vi "FGV_USER_EDITOR_records_display.vi"(4 "front_panel_reference":refnum<vi>, 6 "SQL_listbox_reference":refnum<vi>, 7 "options":T3, 8 "error_in":errorcluster, 10 "uneditable_columns":string[](array[string]), 11 "input":variant) -> (0 "error_out":errorcluster, 1 "all_info":T1, 2 "array_param_output":string[](array[string]), 3 "string_param_output":string)   [LabVIEW 2019]
uses:
  FGV_USER_EDITOR_records_display.ctl
  USER_EDITOR_all_info.ctl
  MAIN/SQL_record_states.ctl
  ini/typedef/CLIENT_all_config_info.ctl
  ini/typedef/CLIENT_main_ini_file.ctl
  queues/typedef/CLIENT_queue_refnums.ctl
  queues/typedef/SQL_EDITOR_queue_element.ctl
  MAIN/SQL_EDITOR/SQL_EDITOR_sequence_state.ctl
  queues/typedef/CLIENT_SCANNER_queue_element.ctl
  MAIN/SCANNER/SCANNER_sequence_state.ctl
  queues/typedef/CLIENT_REF_CHG_queue_element.ctl
  MAIN/reference_changed_connection/CLIENT_REF_CHG_sequence_state.ctl
  login/FGV_login.ctl
  <userlib>/_OpenG.lib/array/array.llb/Filter 1D Array (String)__ogtk.vi
  <userlib>/_OpenG.lib/array/array.llb/Delete Elements from 1D Array (I32)__ogtk.vi
  <vilib>/addons/database/_DB Variant To Data/Database Variant To Data.xnode
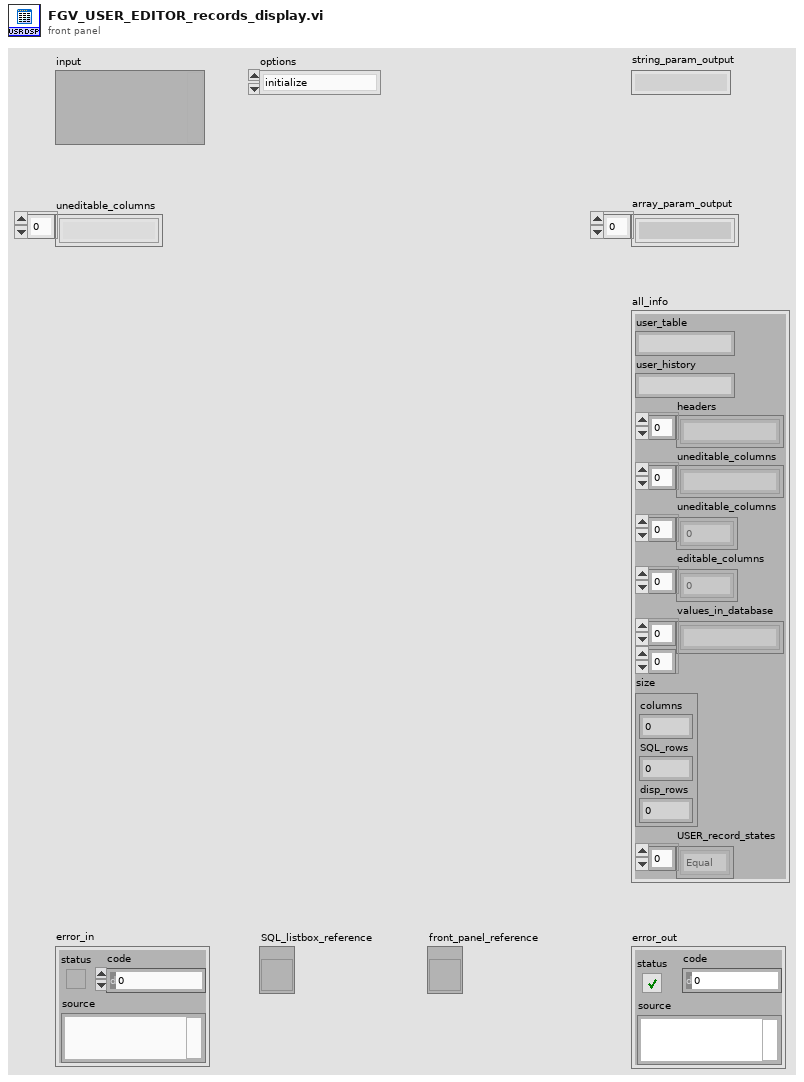
[diagram p1: front panel]
types:
  T1 = typedef "USER_EDITOR_all_info.ctl" = cluster{"user_table":string, "user_history":string, "headers":string[], "uneditable_columns":string[], "uneditable_columns":i32[], "editable_columns":i32[], "values_in_database":string[][], "size":cluster{"columns":i32, "SQL_rows":i32, "disp_rows":i32}, "USER_record_states":T2[]}
  T2 = typedef "SQL_record_states.ctl" = enum16{"Equal", "Added", "Edited", "Deleted"}
  T3 = typedef "FGV_USER_EDITOR_records_display.ctl" = enum16{"initialize", "set_user_edit_tables_names", "set_headers", "set_records", "get_user_edit_table_name", "get_user_edit_hist_table_name", "get_headers", "get_uneditable_columns", "get_all_info", "record_added?", "record_inserted?", "record_edited?", "record_updated?", "record_deleted?", "discard_changes"}
  T4 = typedef "CLIENT_all_config_info.ctl" = cluster{"main_ini_file":T5, "SQL Password":string, "queue_refnums":T6}
  T5 = typedef "CLIENT_main_ini_file.ctl" = cluster{"SQL Driver":string, "SQL Server":string, "SQL Database":string, "SQL UID":string, "Reference table":string, "Reference history":string, "Archivisation CFG table":string, "Archivisation CFG history":string, "User table":string, "User history":string, "logout timeout [ms]":i32, "records per page":i32, "default language":string, "REF CHG connection IP":string, "REF CHG remote port":i32, "REF CHG local port":i32, "SCANNER COM port":u16, "SCANNER Baud rate":u32, "SCANNER Data bits":u16, "SCANNER Pairity":enum16{"None", "Odd", "Even", "Mark", "Space"}, "SCANNER Stop bits":u16, "SCANNER Flow control":u16, "SCANNER Termination char":u8}
  T6 = typedef "CLIENT_queue_refnums.ctl" = cluster{"SQL_EDITOR_queue":refnum<queue>, "SCANNER_queue":refnum<queue>, "SCANNER_data":refnum<queue>, "CLIENT_REF_CHG_queue":refnum<queue>}
  T7 = typedef "FGV_login.ctl" = enum16{"initialize", "login", "logout", "get_login_info"}
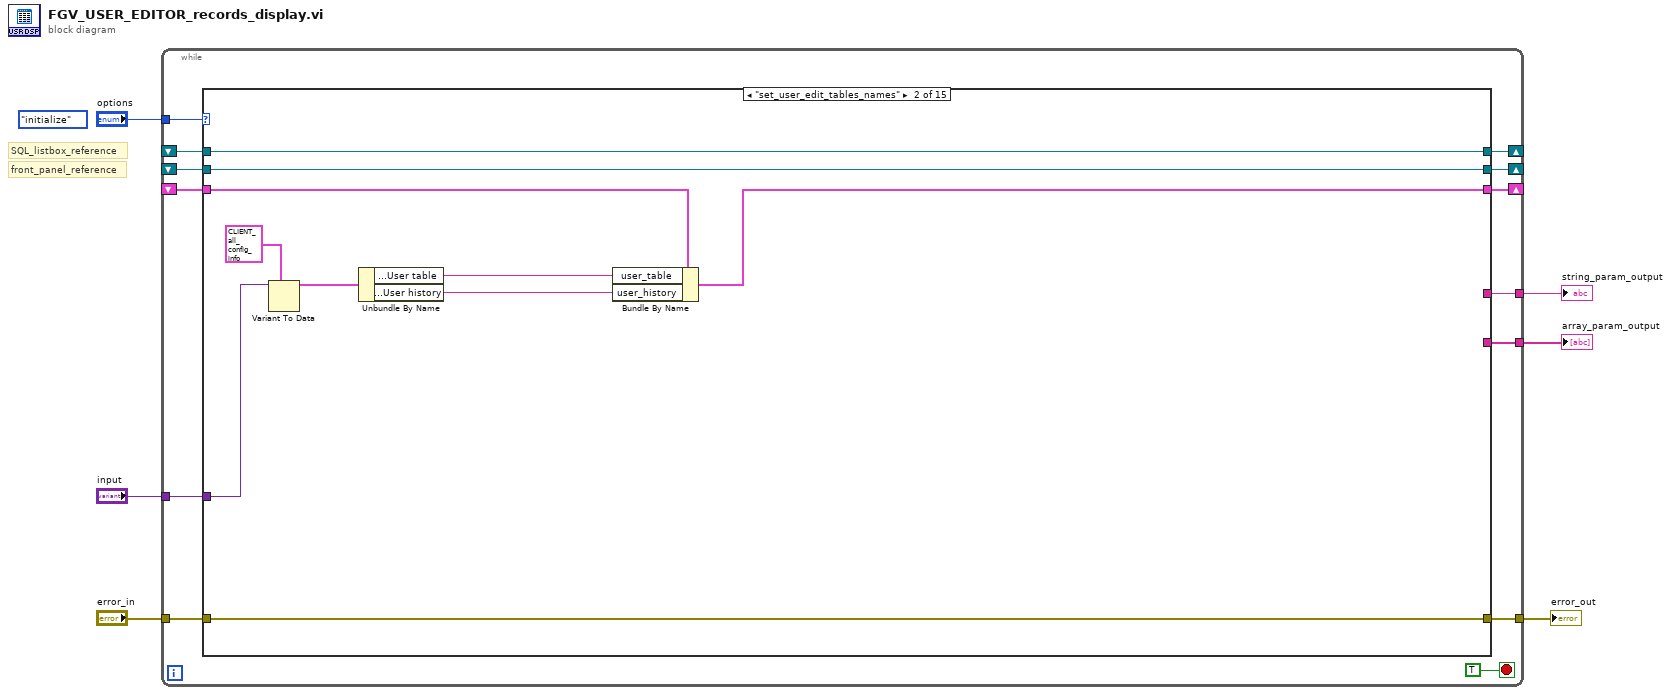
[diagram p0: block diagram]
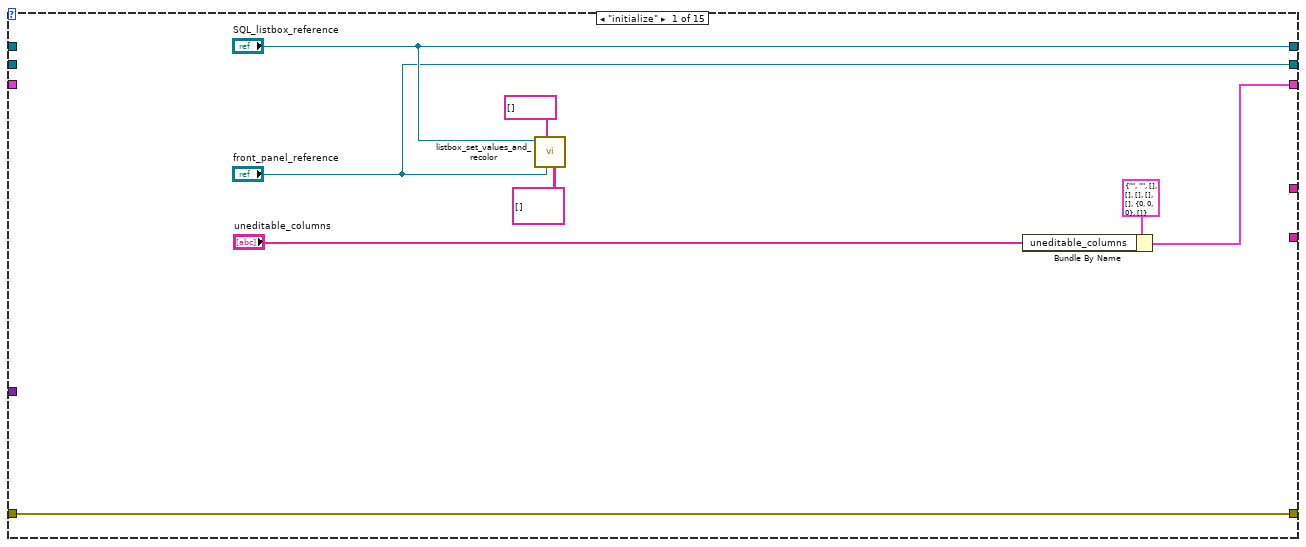
[diagram p2: hidden frame]
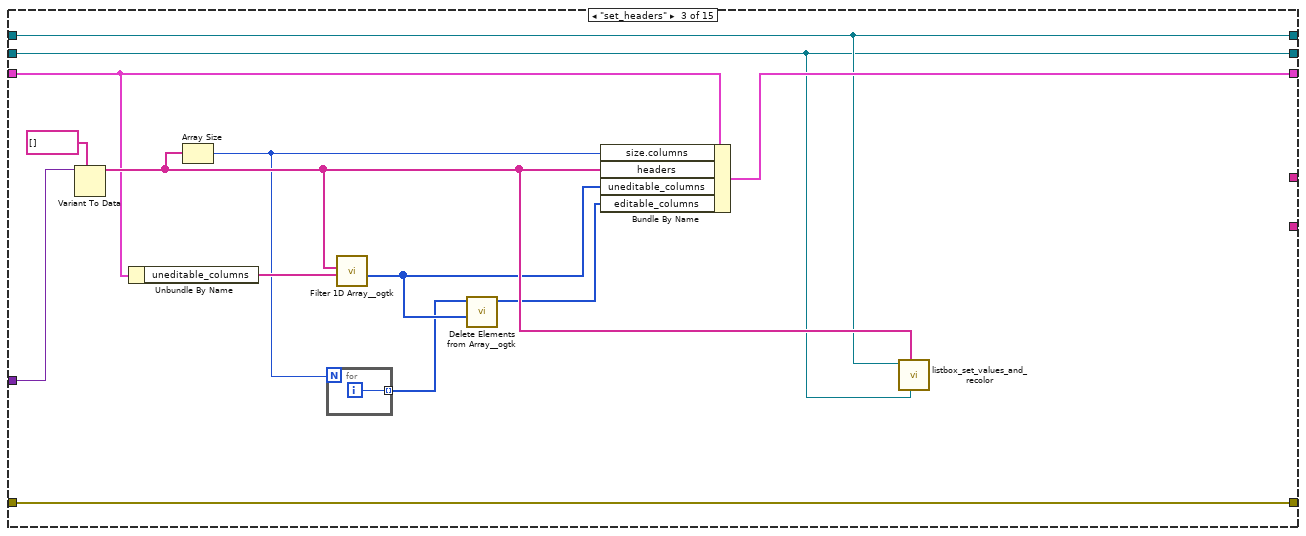
[diagram p3: hidden frame]
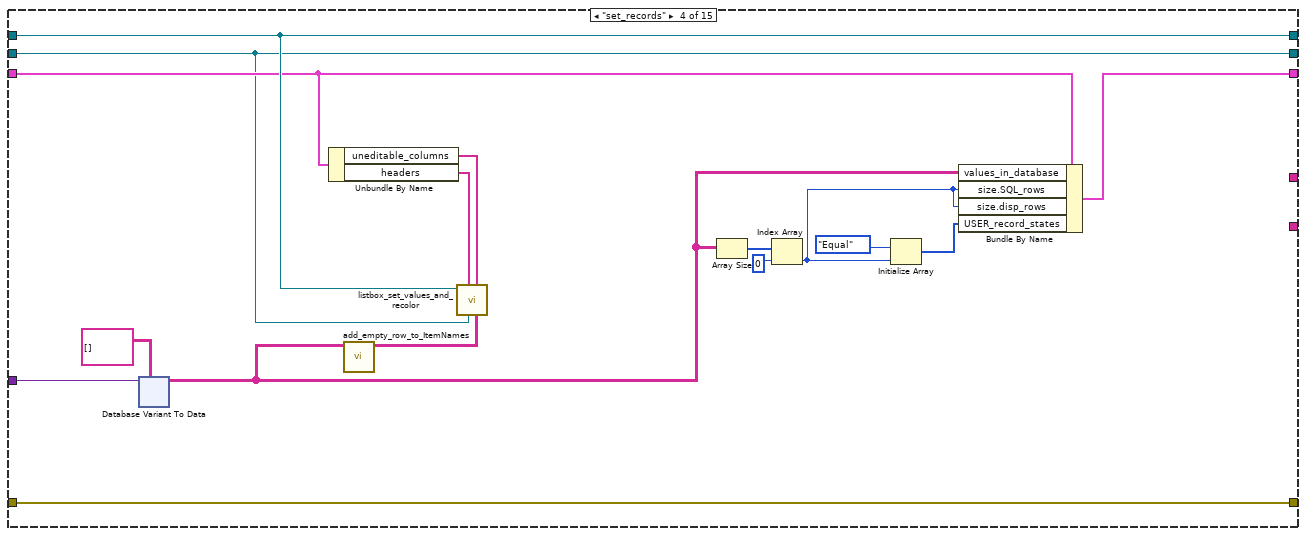
[diagram p4: hidden frame]
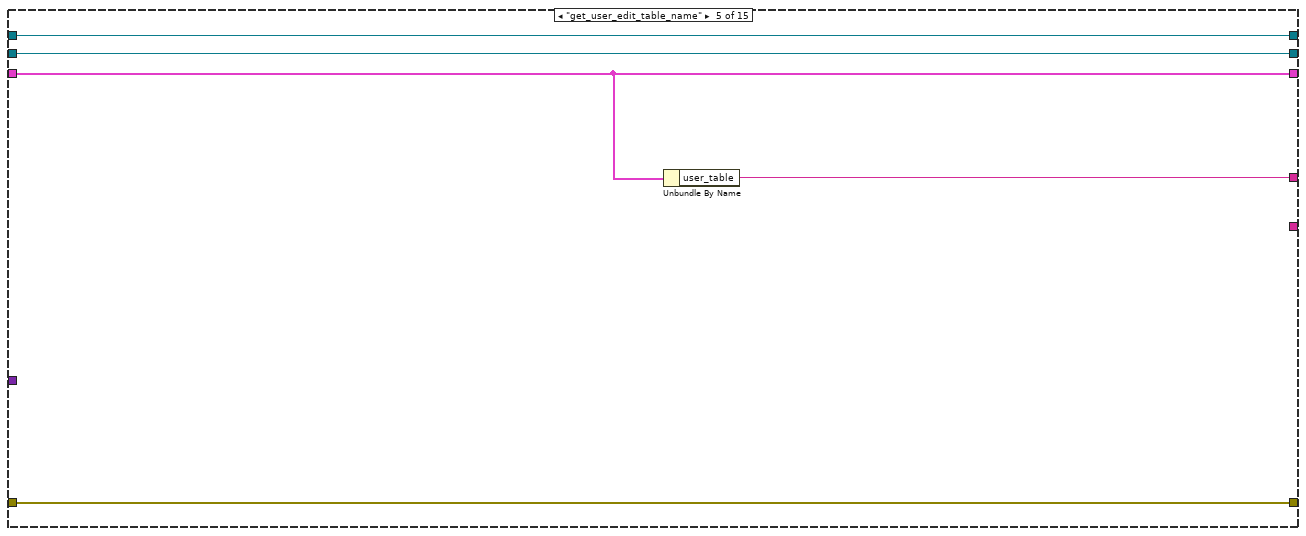
[diagram p5: hidden frame]
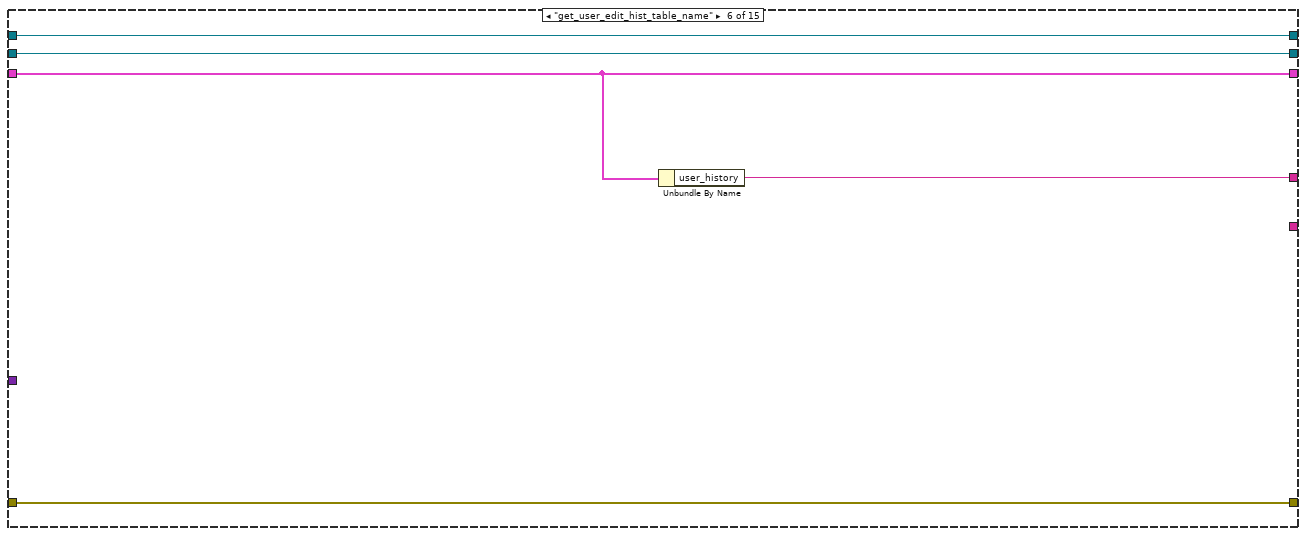
[diagram p6: hidden frame]
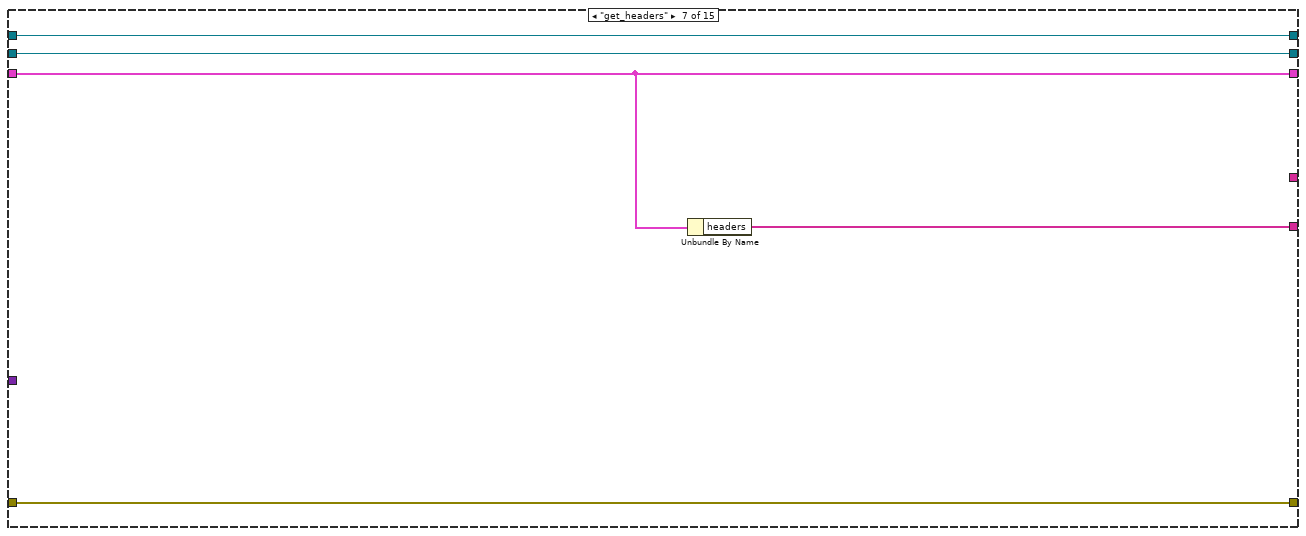
[diagram p7: hidden frame]
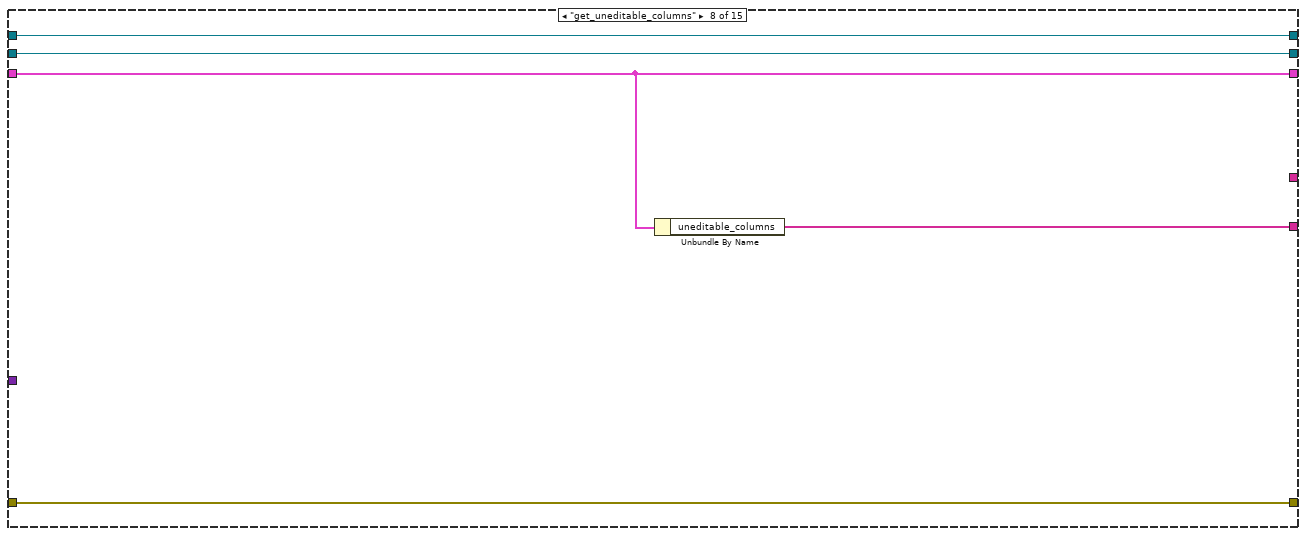
[diagram p8: hidden frame]
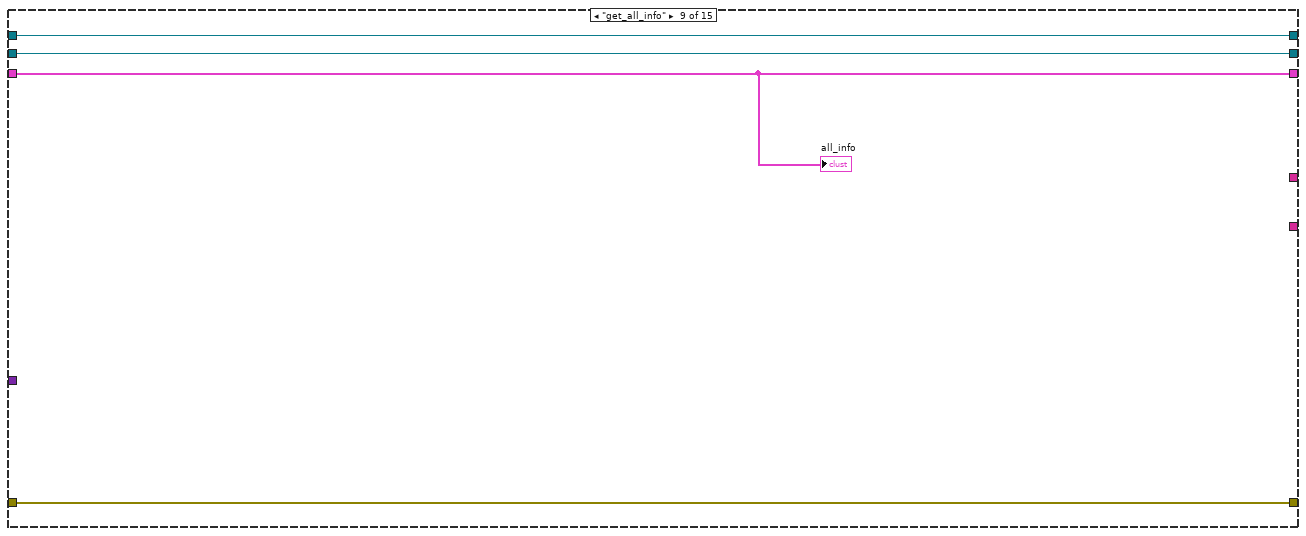
[diagram p9: hidden frame]
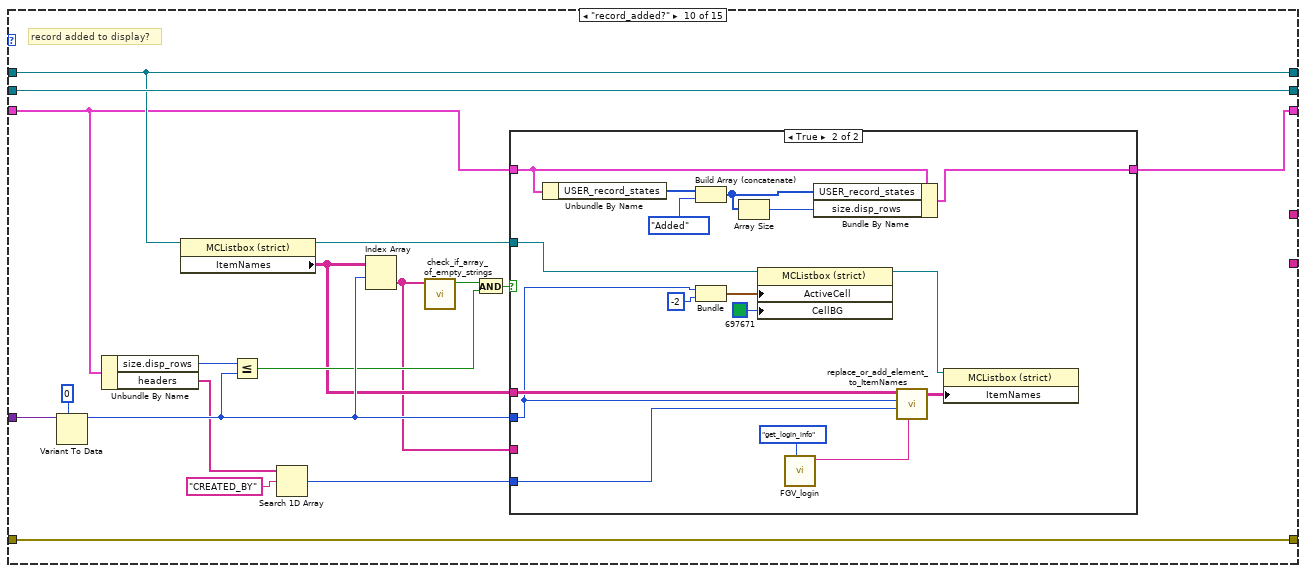
[diagram p10: hidden frame]
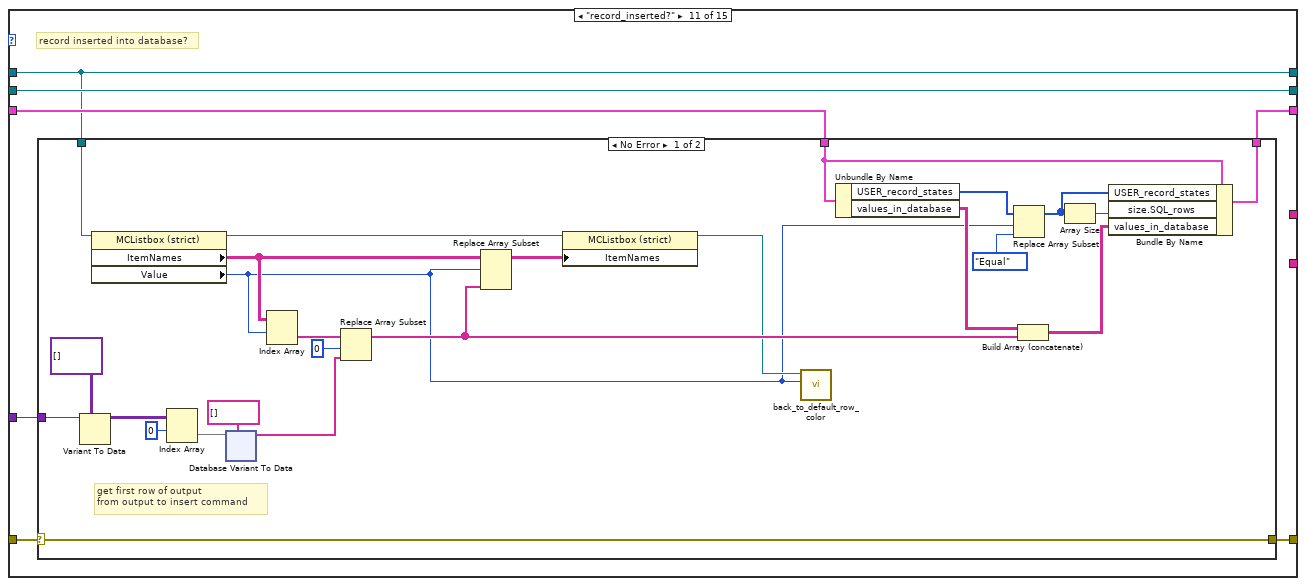
[diagram p12: hidden frame]
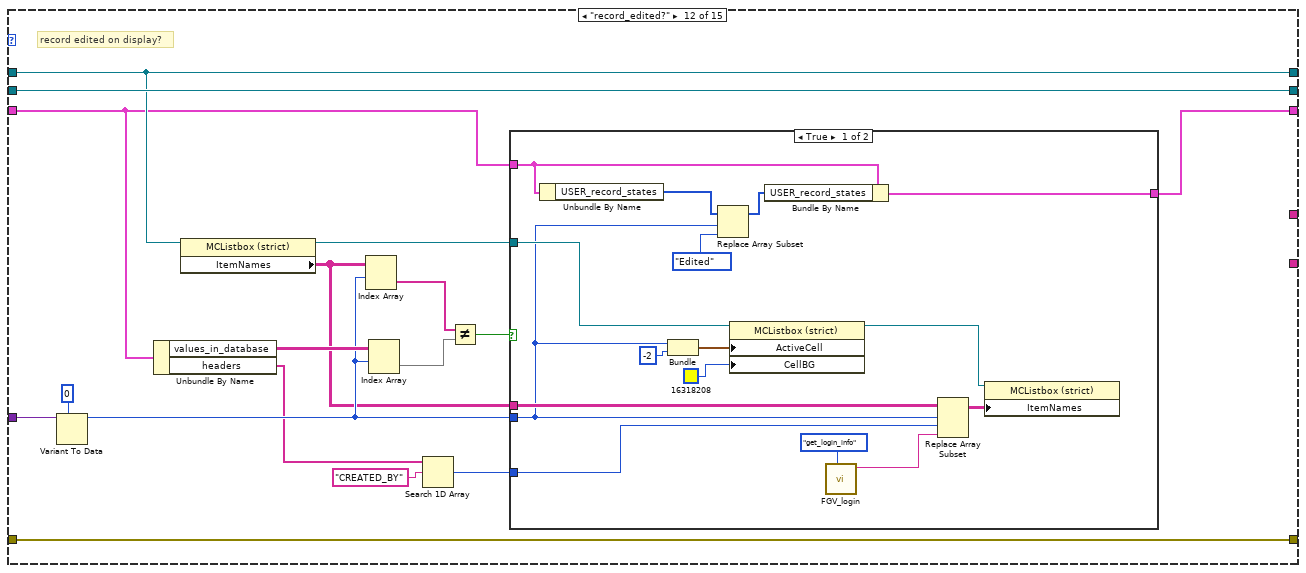
[diagram p14: hidden frame]
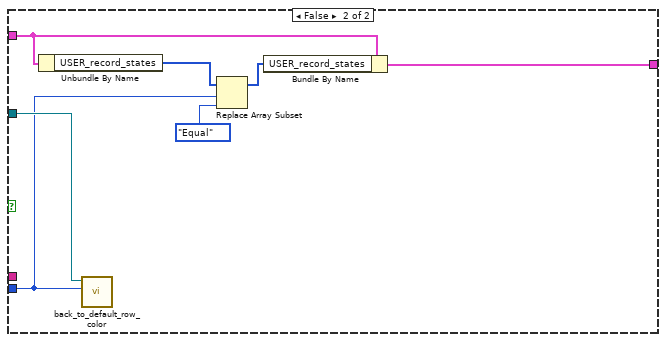
[diagram p15: hidden frame]
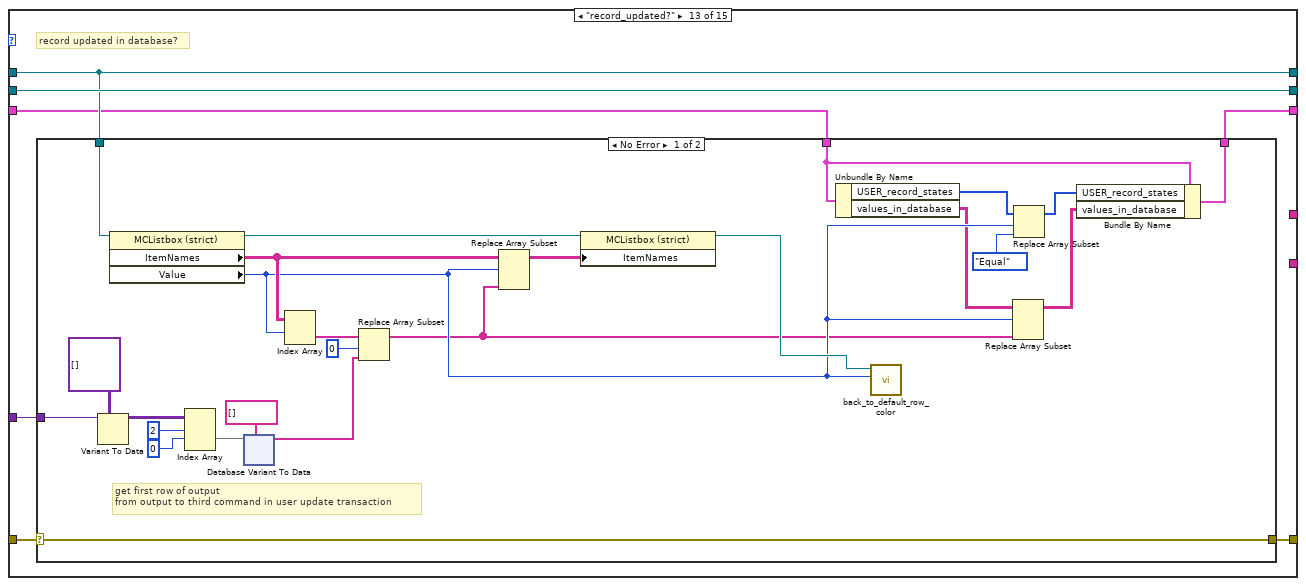
[diagram p16: hidden frame]
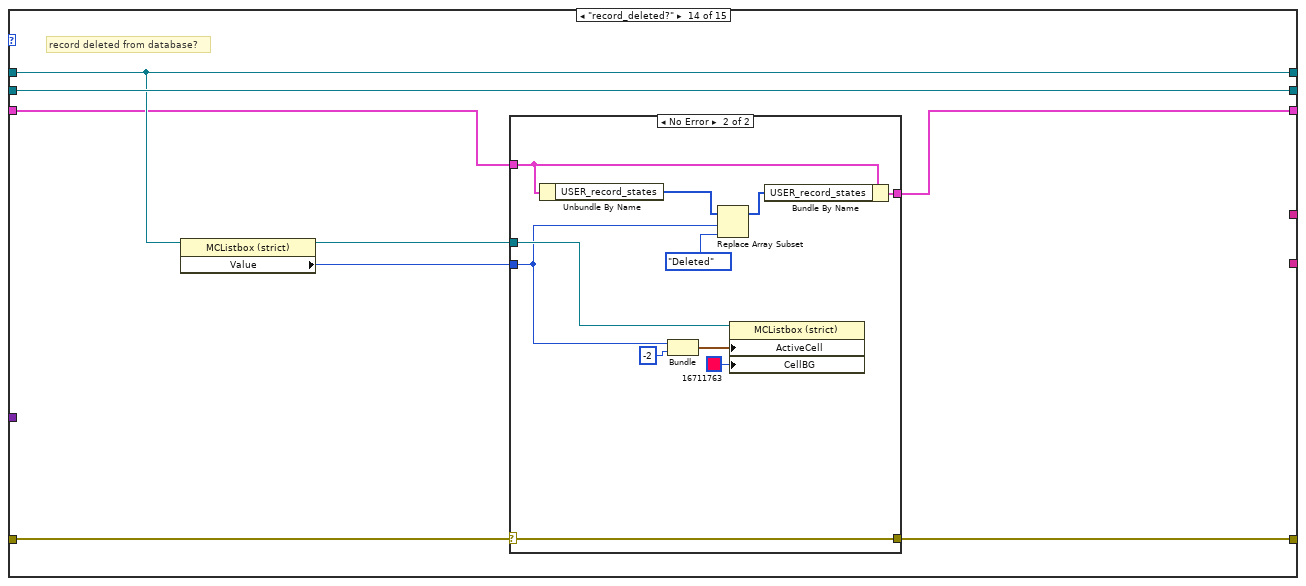
[diagram p18: hidden frame]
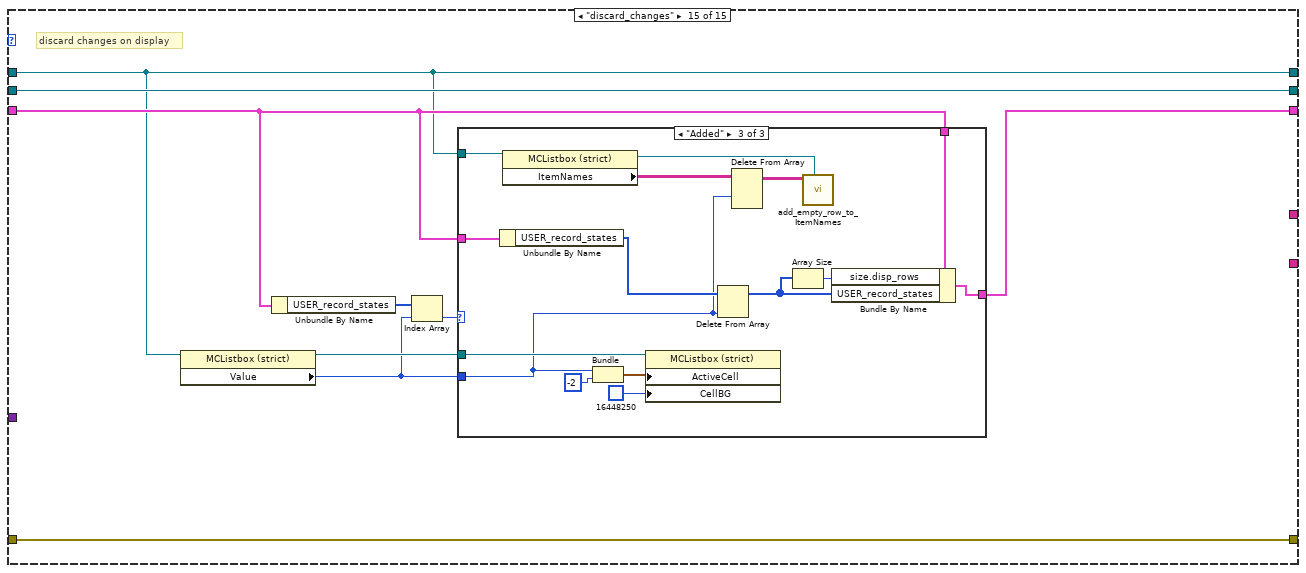
[diagram p20: hidden frame]
diagram:
  (unwired) FGV_USER_EDITOR_records_display."initialize" ("options")
  # "front_panel_reference"
  # "SQL_listbox_reference"
  n1 = while {
    tunnel: "options" -> [w18]
    tunnel: [w17] -> w6
    tunnel: "error_in" -> [w16]
    shift-right: [w15] -> _
    shift-left: _ -> [w14]
    tunnel: [w13] -> w3
    shift-right: [w12] -> _
    shift-left: _ -> [w11]
    tunnel: [w10] -> w2
    tunnel: "input" -> [w9]
    shift-right: [w8] -> _
    shift-left: _ -> [w7]
    stop <- TRUE stop-if-true
    n2 = case shown="\"set_user_edit_tables_names\"" w18 {
      tunnel: [w27 w37 w50 w65 w102 w107 w113 w118 w122 w141 w160 w248 w272 w345 w370] -> w17
      tunnel: w16 -> [w27 w37 w50 w65 w102 w107 w113 w118 w122 w141 w161 w248 w273 w346 w370]
      tunnel: [w23 w35 w40 w61 w104 w109 w114 w119 w123 w135 w164 w236 w275 w347 w371] -> w15
      tunnel: w14 -> [_ w36 w41 w62 w104 w109 w114 w119 w123 w133 w165 w237 w276 w348 w366]
      tunnel: [_ _ _ _ w103 w108 _ _ _ _ _ _ _ _ _] -> w13
      tunnel: ["SQL_listbox_reference" w34 w39 w64 w101 w106 w110 w117 w121 w137 w162 w243 w277 w350 w365] -> w12
      tunnel: w11 -> [_ w34 w39 w64 w101 w106 w110 w117 w121 w137 w162 w243 w277 w350 w365]
      tunnel: [_ _ _ _ _ _ w112 w116 _ _ _ _ _ _ _] -> w10
      tunnel: w9 -> [_ w33 w42 w66 _ _ _ _ _ w139 w163 w246 w274 _ _]
      tunnel: ["front_panel_reference" w32 w38 w54 w100 w105 w111 w115 w120 w140 w166 w247 w278 w351 w373] -> w8
      tunnel: w7 -> [_ w32 w38 w54 w100 w105 w111 w115 w120 w140 w166 w247 w278 w351 w373]
      frame "initialize" {
        n3 = call "listbox_set_values_and_recolor.vi"("item_names"=string[][] [], "front_panel_reference"="front_panel_reference", "column_names"=string[] [], "multicolumn_listbox_reference_in"="SQL_listbox_reference") -> ()  [unwired: 6 in, 2 out]
        n4 = Bundle By Name(cluster=T1 {"user_table"="", "user_history"="", "headers"=[], "uneditable_columns"=[], "uneditable_columns"=[], "editable_columns"=[], "values_in_database"=[], "size"={"columns"=0, "SQL_rows"=0, "disp_rows"=0}, "USER_record_states"=[]} ("SQL_selection"), "uneditable_columns"="uneditable_columns") -> (w23:T1)
      }
      frame "set_user_edit_tables_names" {
        n5 = Variant To Data(type=T4 {"main_ini_file"={"SQL Driver"="", "SQL Server"="", "SQL Database"="", "SQL UID"="", "Reference table"="", "Reference history"="", "Archivisation CFG table"="", "Archivisation CFG history"="", "User table"="", "User history"="", "logout timeout [ms]"=0, "records per page"=0, "default language"="", "REF CHG connection IP"="", "REF CHG remote port"=0, "REF CHG local port"=0, "SCANNER COM port"=0, "SCANNER Baud rate"=0, "SCANNER Data bits"=0, "SCANNER Pairity"=enum."None", "SCANNER Stop bits"=10, "SCANNER Flow control"=0, "SCANNER Termination char"=0}, "SQL Password"="", "queue_refnums"={"SQL_EDITOR_queue"=refnum, "SCANNER_queue"=refnum, "SCANNER_data"=refnum, "CLIENT_REF_CHG_queue"=refnum}} ("all_config_info"), Variant=w33) -> (data=w31:T4)  [unwired: 1 in, 1 out]
        n6 = Unbundle By Name(w31) -> ("main_ini_file.User table"=w30:string, "main_ini_file.User history"=w29:string)
        n7 = Bundle By Name(cluster=w36, "user_table"=w30, "user_history"=w29) -> (w35:T1)
      }
      frame "set_headers" {
        n8 = Variant To Data(type=string[] [], Variant=w42) -> (data=w48:string[])  [unwired: 1 in, 1 out]
        n9 = Unbundle By Name(w41) -> ("uneditable_columns"=w46:string[])
        n10 = Array Size(array=w48) -> (size(s)=w43:i32)
        n11 = for {
          N: w43 -> [_]
          tunnel: [w51] -> w45 mode=indexing
          i -> [w51]
        }
        n12 = call-poly <userlib>:"Filter 1D Array__ogtk.vi"("items to filter"=w46, "array"=w48) -> ("filtered item indices"=w47:i32[])  [unwired: 4 in, 1 out]
        n13 = call-poly <userlib>:"Delete Elements from Array__ogtk.vi"("indices"=w47, "array"=w45) -> ("array w/ subset deleted"=w44:i32[])  [unwired: 8 in, 1 out]
        n14 = Bundle By Name(cluster=w41, "size.columns"=w43, "headers"=w48, "uneditable_columns"=w47, "editable_columns"=w44) -> (w40:T1)
        n15 = call "listbox_set_values_and_recolor.vi"("front_panel_reference"=w38, "column_names"=w48, "multicolumn_listbox_reference_in"=w39) -> ()  [unwired: 7 in, 2 out]
      }
      frame "set_records" {
        n16 = xnode "Database Variant To Data"("database variant"=w66, "type"=string[][] []) -> ("data"=w52:string[][])  [unwired: 1 in, 1 out]
        n17 = Unbundle By Name(w62) -> ("uneditable_columns"=w55:string[], "headers"=w63:string[])
        n18 = call "add_empty_row_to_ItemNames.vi"("ItemNames_in"=w52) -> ("ItemNames_out"=w53:string[][])  [unwired: 10 in]
        n19 = call "listbox_set_values_and_recolor.vi"("item_names"=w53, "uneditable_columns"=w55, "front_panel_reference"=w54, "column_names"=w63, "multicolumn_listbox_reference_in"=w64) -> ()  [unwired: 5 in, 2 out]
        n20 = Array Size(array=w52) -> (size(s)=w60:i32[])
        n21 = Index Array(array=w60, index=0) -> (element=w57:i32)
        n22 = Initialize Array(SQL_record_states."Equal", w57) -> (w56:T2[])
        n23 = Bundle By Name(cluster=w62, "values_in_database"=w52, "size.SQL_rows"=w57, "size.disp_rows"=w57, "USER_record_states"=w56) -> (w61:T1)
      }
      frame "get_user_edit_table_name" {
        n24 = Unbundle By Name(w104) -> ("user_table"=w103:string)
      }
      frame "get_user_edit_hist_table_name" {
        n25 = Unbundle By Name(w109) -> ("user_history"=w108:string)
      }
      frame "get_headers" {
        n26 = Unbundle By Name(w114) -> ("headers"=w112:string[])
      }
      frame "get_uneditable_columns" {
        n27 = Unbundle By Name(w119) -> ("uneditable_columns"=w116:string[])
      }
      frame "get_all_info" {
        "all_info" <- w123
      }
      frame "record_added?" {
        # "record added to display?"
        n28 = Variant To Data(type=0, Variant=w139) -> (data=w131:i32)  [unwired: 1 in, 1 out]
        n29 = Unbundle By Name(w133) -> ("size.disp_rows"=w132:i32, "headers"=w128:string[])
        n30 = property class="MCListbox (strict)"(reference=w137) -> (reference out=w136:refnum<vi>, "ItemNames"=w129:string[][])  [unwired: 1 in, 1 out]
        n31 = Less Or Equal?(x=w132, y=w131) -> (x <= y?=w130:bool)
        n32 = Search 1D Array(1D array=w128, element="CREATED_BY") -> (index of element=w126:i32)  [unwired: 1 in]
        n33 = Index Array(array=w129, index (row)=w131) -> (element=w125:string[])  [unwired: 1 in]
        n34 = call "check_if_array_of_empty_strings.vi"("array"=w125) -> ("Not empty?"=w124:bool)  [unwired: 10 in]
        n35 = And(x=w124, y=w130) -> (x .and. y?=w134:bool)
        n36 = case shown="True" w134 {
          tunnel: w131 -> [_ w147]
          tunnel: w136 -> [_ w156]
          tunnel: w133 -> [w142 w154]
          tunnel: [w142 w155] -> w135
          tunnel: w129 -> [_ w148]
          tunnel: w125 -> [_ _]
          tunnel: w126 -> [_ w146]
          frame False {
          }
          frame True {
            n37 = Unbundle By Name(w154) -> ("USER_record_states"=w153:T2[])
            n38 = Build Array (concatenate)(w153, SQL_record_states."Added" ("new element/subarray")) -> (w151:T2[])
            n39 = Bundle(w147, -2) -> (w157:cluster{i32, i32})  [unwired: 1 in]
            n40 = Array Size(array=w151) -> (size(s)=w150:i32)
            n41 = property on="Property Node" class="MCListbox (strict)"(reference=w156, "ActiveCell"=w157, "CellBG"=u32 697671) -> (reference out=w145:refnum<vi>)  [unwired: 1 in, 1 out]
            n42 = call "FGV_login.vi"("options"=FGV_login."get_login_info") -> ("username_out"=w143:string)  [unwired: 8 in, 2 out]
            n43 = Bundle By Name(cluster=w154, "USER_record_states"=w151, "size.disp_rows"=w150) -> (w155:T1)
            n44 = call "replace_or_add_element_to_ItemNames.vi"("element"=w143, "column"=w146, "row"=w147, "ItemNames_in"=w148) -> ("ItemNames_out"=w149:string[][])  [unwired: 7 in]
            n45 = property class="MCListbox (strict)"(reference=w145, "ItemNames"=w149) -> ()  [unwired: 1 in, 2 out]
          }
        }
      }
      frame "record_inserted?" {
        # "record inserted into database?"
        n46 = case shown="No Error" w161 {
          selector: w161 -> [w167 w231]
          tunnel: w165 -> [w191 w230]
          tunnel: [w190 w230] -> w164
          tunnel: w163 -> [w173 _]
          tunnel: w162 -> [w172 _]
          tunnel: [w167 w231] -> w160
          frame No Error {
            # "get first row of output\nfrom output to insert command"
            n47 = Variant To Data(type=variant[][] [], Variant=w173) -> (data=w182:variant[][])  [unwired: 1 in, 1 out]
            n48 = property class="MCListbox (strict)"(reference=w172) -> (reference out=w176:refnum<vi>, "ItemNames"=w175:string[][], "Value"=w169:i32)  [unwired: 1 in, 1 out]
            n49 = Index Array(array=w182, index (row)=0) -> (element=w179:variant[])  [unwired: 1 in]
            n50 = xnode "Database Variant To Data"("database variant"=w179, "type"=string[] []) -> ("data"=w177:string[])  [unwired: 1 in, 1 out]
            n51 = Index Array(array=w175, index (row)=w169) -> (element=w181:string[])  [unwired: 1 in]
            n52 = Replace Array Subset(array=w181, new element=w177, index=0) -> (w171:string[])
            n53 = Replace Array Subset(array=w175, new element=w171, index (row)=w169) -> (w174:string[][])  [unwired: 1 in]
            n54 = property class="MCListbox (strict)"(reference=w176, "ItemNames"=w174) -> (reference out=w170:refnum<vi>)  [unwired: 1 in, 1 out]
            n55 = call "back_to_default_row_color.vi"("row"=w169, "listbox_reference"=w170) -> ()  [unwired: 9 in, 1 out]
            n56 = Unbundle By Name(w191) -> ("USER_record_states"=w188:T2[], "values_in_database"=w187:string[][])
            n57 = Replace Array Subset(array=w188, new element=SQL_record_states."Equal" ("new element/subarray"), index=w169) -> (w184:T2[])
            n58 = Build Array (concatenate)(w187, w171) -> (w186:string[][])
            n59 = Array Size(array=w184) -> (size(s)=w185:i32)
            n60 = Bundle By Name(cluster=w191, "USER_record_states"=w184, "size.SQL_rows"=w185, "values_in_database"=w186) -> (w190:T1)
          }
          frame Error {
          }
        }
      }
      frame "record_edited?" {
        # "record edited on display?"
        n61 = Variant To Data(type=0, Variant=w246) -> (data=w238:i32)  [unwired: 1 in, 1 out]
        n62 = Unbundle By Name(w237) -> ("values_in_database"=w244:string[][], "headers"=w233:string[])
        n63 = property class="MCListbox (strict)"(reference=w243) -> (reference out=w239:refnum<vi>, "ItemNames"=w235:string[][])  [unwired: 1 in, 1 out]
        n64 = Index Array(array=w235, index (row)=w238) -> (element=w242:string[])  [unwired: 1 in]
        n65 = Index Array(array=w244, index (row)=w238) -> (element=w241:string[])  [unwired: 1 in]
        n66 = Search 1D Array(1D array=w233, element="CREATED_BY") -> (index of element=w232:i32)  [unwired: 1 in]
        n67 = Not Equal?(x=w242, y=w241) -> (x != y?=w240:bool)
        n68 = case shown="True" w240 {
          tunnel: w238 -> [w250 w265]
          tunnel: w239 -> [w262 w266]
          tunnel: w237 -> [w258 w269]
          tunnel: [w256 w267] -> w236
          tunnel: w235 -> [w251 _]
          tunnel: w232 -> [w249 _]
          frame True {
            n69 = Unbundle By Name(w258) -> ("USER_record_states"=w259:T2[])
            n70 = Bundle(w250, -2) -> (w263:cluster{i32, i32})  [unwired: 1 in]
            n71 = Replace Array Subset(array=w259, new element=SQL_record_states."Edited" ("new element/subarray"), index=w250) -> (w257:T2[])
            n72 = property on="Property Node" class="MCListbox (strict)"(reference=w262, "ActiveCell"=w263, "CellBG"=u32 16318208) -> (reference out=w252:refnum<vi>)  [unwired: 1 in, 1 out]
            n73 = Bundle By Name(cluster=w258, "USER_record_states"=w257) -> (w256:T1)
            n74 = call "FGV_login.vi"("options"=FGV_login."get_login_info") -> ("username_out"=w253:string)  [unwired: 8 in, 2 out]
            n75 = Replace Array Subset(array=w251, new element=w253, index (row)=w250, index (col)=w249) -> (w255:string[][])
            n76 = property class="MCListbox (strict)"(reference=w252, "ItemNames"=w255) -> ()  [unwired: 1 in, 2 out]
          }
          frame False {
            n77 = Unbundle By Name(w269) -> ("USER_record_states"=w270:T2[])
            n78 = call "back_to_default_row_color.vi"("row"=w265, "listbox_reference"=w266) -> ()  [unwired: 9 in, 1 out]
            n79 = Replace Array Subset(array=w270, new element=SQL_record_states."Equal" ("new element/subarray"), index=w265) -> (w268:T2[])
            n80 = Bundle By Name(cluster=w269, "USER_record_states"=w268) -> (w267:T1)
          }
        }
      }
      frame "record_updated?" {
        # "record updated in database?"
        n81 = case shown="No Error" w273 {
          selector: w273 -> [w279 w342]
          tunnel: w277 -> [w303 _]
          tunnel: w276 -> [w302 w343]
          tunnel: [w301 w343] -> w275
          tunnel: w274 -> [w300 _]
          tunnel: [w279 w342] -> w272
          frame No Error {
            # "get first row of output\nfrom output to third command in user update transaction"
            n82 = Variant To Data(type=variant[][][] [], Variant=w300) -> (data=w298:variant[][][])  [unwired: 1 in, 1 out]
            n83 = property class="MCListbox (strict)"(reference=w303) -> (reference out=w290:refnum<vi>, "ItemNames"=w288:string[][], "Value"=w286:i32)  [unwired: 1 in, 1 out]
            n84 = Index Array(array=w298, index (dim 0)=2 ("index (page)"), index (dim 1)=0 ("disabled index (row)")) -> (element=w293:variant[])  [unwired: 1 in]
            n85 = xnode "Database Variant To Data"("database variant"=w293, "type"=string[] []) -> ("data"=w291:string[])  [unwired: 1 in, 1 out]
            n86 = Index Array(array=w288, index (row)=w286) -> (element=w295:string[])  [unwired: 1 in]
            n87 = Replace Array Subset(array=w295, new element=w291, index=0) -> (w285:string[])
            n88 = Replace Array Subset(array=w288, new element=w285, index (row)=w286) -> (w287:string[][])  [unwired: 1 in]
            n89 = property class="MCListbox (strict)"(reference=w290, "ItemNames"=w287) -> (reference out=w289:refnum<vi>)  [unwired: 1 in, 1 out]
            n90 = Unbundle By Name(w302) -> ("USER_record_states"=w283:T2[], "values_in_database"=w280:string[][])
            n91 = call "back_to_default_row_color.vi"("row"=w286, "listbox_reference"=w289) -> ()  [unwired: 9 in, 1 out]
            n92 = Replace Array Subset(array=w280, new element=w285, index (row)=w286) -> (w281:string[][])  [unwired: 1 in]
            n93 = Replace Array Subset(array=w283, new element=SQL_record_states."Equal" ("new element/subarray"), index=w286) -> (w282:T2[])
            n94 = Bundle By Name(cluster=w302, "USER_record_states"=w282, "values_in_database"=w281) -> (w301:T1)
          }
          frame Error {
          }
        }
      }
      frame "record_deleted?" {
        # "record deleted from database?"
        n95 = property class="MCListbox (strict)"(reference=w350) -> (reference out=w349:refnum<vi>, "Value"=w344:i32)  [unwired: 1 in, 1 out]
        n96 = case shown="No Error" w346 {
          selector: w346 -> [w353 w354]
          tunnel: w349 -> [_ w362]
          tunnel: w348 -> [w352 w358]
          tunnel: [w352 w356] -> w347
          tunnel: [w353 w354] -> w345
          tunnel: w344 -> [_ w355]
          frame Error {
          }
          frame No Error {
            n97 = Unbundle By Name(w358) -> ("USER_record_states"=w359:T2[])
            n98 = Bundle("Value"=w355, -2) -> (w363:cluster{"Value":i32, i32})  [unwired: 1 in]
            n99 = Replace Array Subset(array=w359, new element=SQL_record_states."Deleted" ("new element/subarray"), index=w355) -> (w357:T2[])
            n100 = property on="Property Node" class="MCListbox (strict)"(reference=w362, "ActiveCell"=w363, "CellBG"=u32 16711763) -> ()  [unwired: 1 in, 2 out]
            n101 = Bundle By Name(cluster=w358, "USER_record_states"=w357) -> (w356:T1)
          }
        }
      }
      frame "discard_changes" {
        # "discard changes on display"
        n102 = property class="MCListbox (strict)"(reference=w365) -> (reference out=w372:refnum<vi>, "Value"=w368:i32)  [unwired: 1 in, 1 out]
        n103 = Unbundle By Name(w366) -> ("USER_record_states"=w369:T2[])
        n104 = Index Array(array=w369, index=w368) -> (element=w367:T2)
        n105 = case shown="\"Added\"" w367 {
          tunnel: w372 -> [_ w388 w394]
          tunnel: w366 -> [w374 w387 w403]
          tunnel: [w374 w386 w402] -> w371
          tunnel: w368 -> [_ w378 w393]
          tunnel: w366 -> [_ w383 w401]
          tunnel: w365 -> [_ w381 w399]
          frame Default {
          }
          frame "Edited" {
            n106 = Unbundle By Name(w383) -> ("values_in_database"=w379:string[][], "USER_record_states"=w382:T2[])
            n107 = property class="MCListbox (strict)"(reference=w381) -> (reference out=w376:refnum<vi>, "ItemNames"=w380:string[][])  [unwired: 1 in, 1 out]
            n108 = call "back_to_default_row_color.vi"("row"=w378, "listbox_reference"=w388) -> ()  [unwired: 9 in, 1 out]
            n109 = Index Array(array=w379, index (row)=w378) -> (element=w377:string[])  [unwired: 1 in]
            n110 = Replace Array Subset(array=w382, new element=SQL_record_states."Equal" ("new element/subarray"), index=w378) -> (w384:T2[])
            n111 = Replace Array Subset(array=w380, new element=w377, index (row)=w378) -> (w375:string[][])  [unwired: 1 in]
            n112 = property class="MCListbox (strict)"(reference=w376, "ItemNames"=w375) -> ()  [unwired: 1 in, 2 out]
            n113 = Bundle By Name(cluster=w387, "USER_record_states"=w384) -> (w386:T1)
          }
          frame "Added" {
            n114 = Unbundle By Name(w401) -> ("USER_record_states"=w400:T2[])
            n115 = property class="MCListbox (strict)"(reference=w399) -> (reference out=w389:refnum<vi>, "ItemNames"=w398:string[][])  [unwired: 1 in, 1 out]
            n116 = Bundle("Value"=w393, -2) -> (w397:cluster{"Value":i32, i32})  [unwired: 1 in]
            n117 = property on="Property Node" class="MCListbox (strict)"(reference=w394, "ActiveCell"=w397, "CellBG"=u32 16448250) -> ()  [unwired: 1 in, 2 out]
            n118 = Delete From Array(array=w400, index=w393) -> (array with subset deleted=w391:T2[])  [unwired: 1 in, 1 out]
            n119 = Delete From Array(array=w398, index (row)=w393) -> (array with subset deleted=w390:string[][])  [unwired: 2 in, 1 out]
            n120 = Array Size(array=w391) -> (size(s)=w392:i32)
            n121 = call "add_empty_row_to_ItemNames.vi"("multicolumn_listbox_reference_in"=w389, "ItemNames_in"=w390) -> ()  [unwired: 9 in, 1 out]
            n122 = Bundle By Name(cluster=w403, "size.disp_rows"=w392, "USER_record_states"=w391) -> (w402:T1)
          }
        }
      }
    }
  }
  "error_out" <- w6
  "string_param_output" <- w3
  "array_param_output" <- w2
